vi "Received Pressure.vi"(8 "error in (no error)":errorcluster, 10 "Received Pressure":waveform(dbl), 11 "Pressure Gauges in":refnum<class "Pressure Gauges.lvclass">) -> (0 "error out":errorcluster, 3 "Pressure Gauges out":refnum<class "Pressure Gauges.lvclass">)   [LabVIEW 2021, in "Pressure Gauges.lvclass"]
uses:
  Pressure Gauges.lvclass
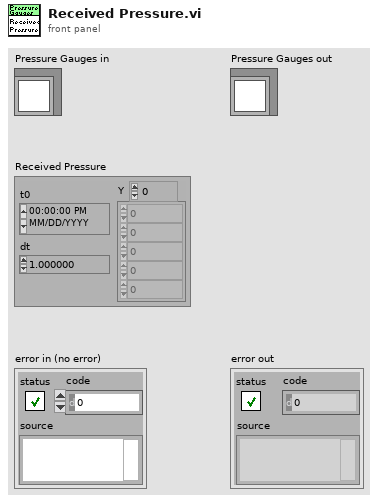
[diagram p1: front panel]
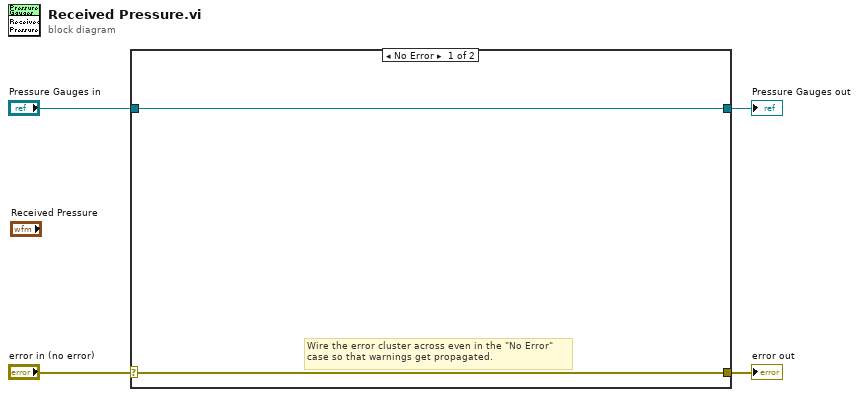
[diagram p0: block diagram]
diagram:
  n1 = case shown="No Error" "error in (no error)" {
    selector: "error in (no error)" -> [w5 w8]
    tunnel: [w5 w8] -> w3
    tunnel: [w6 w7] -> w1
    tunnel: "Pressure Gauges in" -> [w6 w7]
    frame No Error {
      # "Wire the error cluster across even in the \"No Error\"\ncase so that warnings get propagated."
    }
    frame Error {
    }
  }
  "error out" <- w3
  "Pressure Gauges out" <- w1
